vi "Shut_down_all_Axis.vi"   [LabVIEW 2010]
uses:
  GenericDriveCommand.ctl
  DriveConfigGlobal.vi
types:
  T1 = typedef "AxisConfigCluster.ctl" = cluster{"Channel Properties":T2, "Static Drive Configuration":T3}
  T2 = typedef "DriveProperties.ctl" = cluster{"Channel Name":string, "Vel. Default":dbl, "Acc. Default":dbl, "Vel. Max":dbl, "Vel. Min":dbl, "Acc. Max":dbl, "Acc. Min":dbl, "Pulses/unit":dbl, "Address":u8, "Pulse Offset":i32, "Pos Tolerance":dbl, "Pulses/rev":dbl, "Backlash/Eng units":dbl, "Current Pos":dbl, "Ch Status":enum16{"Active", "Offline", "Simulate"}, "Port Name":string, "Axis Transform mode":string, "Metadata Ch Name":string, "Type":string}
  T3 = typedef "DriveStaticConfig.ctl" = cluster{"Correction Gain % (CG)":u16, "Dead Band (DB)":i32, "Dead Band Window (DW)":i32, "Encoder Resolution (ER)":i32, "Step Mode  (FSB)":u16, "Position Maintenance (FSC)":u16, "Stop on Stall (FSD)":u16, "Activate OP1 on stall (FSE)":u16, "Stop on Trigger 3 (FSF)":u16, "OP2 in Deadband (FSG)":u16, "Stall Detect (FSH)":u16, "Limit Disable (LD)":u16, "Motor Resolution (MR)":enum16{"200", "400", "1000", "2000", "4000", "5000", "10000", "12800", "18000", "20000", "21600", "25000", "25400", "25600", "36000", "50000", "278528", "425984", "507904", "614400", "655360", "819200", "1024000"}, "Limit Switch Sense (OSA)":u16, "Home Position (OSB)":u16, "Home Switch Sense (OSC)":u16, "Encoder Z for Home (OSD)":u16, "Reference edge of Home (OSH)":u16, "RS232 Echo Control (SSA)":u16, "Buffer at Limit (SSG)":u16, "Buffer at Stop (SSH)":u16, "Indexer Mode  (FSA)":u16, "Type":string, "ConfigString":string, "De Power Motor":enum16{"TRUE", "FALSE"}}
  T4 = typedef "GenericDriveCommand.ctl" = string
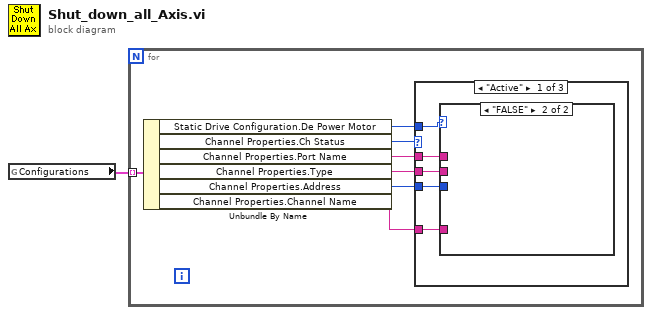
[diagram p0: block diagram]
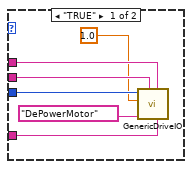
[diagram p2: hidden frame]
diagram:
  n1 = global read "DriveConfigGlobal.vi" "Configurations"() -> (w1:T1[])
  n2 = for {
    tunnel: w1 -> [w8] mode=indexing
    n3 = Unbundle By Name(w8) -> ("Static Drive Configuration.De Power Motor"=w2:enum16{"TRUE", "FALSE"}, "Channel Properties.Ch Status"=w7:enum16{"Active", "Offline", "Simulate"}, "Channel Properties.Port Name"=w6:string, "Channel Properties.Type"=w5:string, "Channel Properties.Address"=w4:u8, "Channel Properties.Channel Name"=w3:string)
    n4 = case shown="\"Active\"" w7 {
      tunnel: w6 -> [w13 _ _]
      tunnel: w5 -> [w12 _ _]
      tunnel: w4 -> [w11 _ _]
      tunnel: w3 -> [w10 _ _]
      tunnel: w2 -> [w9 _ _]
      frame "Active" {
        n5 = case shown="\"FALSE\"" w9 {
          tunnel: w13 -> [w19 _]
          tunnel: w12 -> [w18 _]
          tunnel: w11 -> [w17 _]
          tunnel: w10 -> [w16 _]
          frame "TRUE" {
            n6 = call "GenericDriveIO.vi"("GenericDriveCommand"=T4 "DePowerMotor", "Channel Name"=w16, "Numeric Value"=1.0, "Address"=w17, "Type"=w18, "Port Name"=w19) -> ()  [unwired: 1 in, 5 out]
          }
          frame "FALSE" {
          }
        }
      }
      frame "Offline" {
      }
      frame "Simulate" {
      }
    }
  }
